vi "Strings to Helium Configuration.vi"(10 "Thresholds":string[][](array[string]), 11 "Timings":string[][](array[string])) -> (2 "Thresholds":T1[](array[typedef]), 3 "Timings":T2[](array[typedef]))   [LabVIEW 2015]
uses:
  Tests/Controls/Test Timing.ctl
  Tests/Controls/Helium Thresholds.ctl
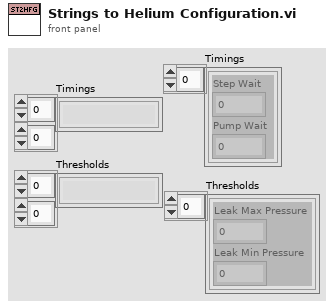
[diagram p1: front panel]
types:
  T1 = typedef "Helium Thresholds.ctl" = cluster{"Leak Max Pressure":dbl, "Leak Min Pressure":dbl}
  T2 = typedef "Test Timing.ctl" = cluster{"Step Wait":dbl, "Pump Wait":dbl}
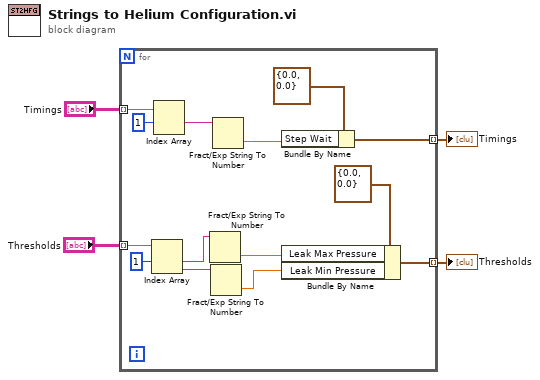
[diagram p0: block diagram]
diagram:
  n1 = for {
    tunnel: "Timings" -> [w18] mode=indexing
    tunnel: "Thresholds" -> [w14] mode=indexing
    tunnel: [w8] -> w2 mode=indexing
    tunnel: [w7] -> w1 mode=indexing
    n2 = Index Array(array=w14, index #1=1 ("index")) -> (element #1=w12:string, element #2=w11:string)  [unwired: 1 in]
    n3 = Index Array(array=w18, index #1=1 ("index")) -> (element #1=w16:string)  [unwired: 1 in, 1 out]
    n4 = Fract/Exp String To Number(string=w12) -> (number=w10:dbl)  [unwired: 3 in, 1 out]
    n5 = Fract/Exp String To Number(string=w11) -> (number=w9:dbl)  [unwired: 3 in, 1 out]
    n6 = Fract/Exp String To Number(string=w16) -> (number=w15:dbl)  [unwired: 3 in, 1 out]
    n7 = Bundle By Name(cluster=T2 {"Step Wait"=0.0, "Pump Wait"=0.0} ("Timing"), "Step Wait"=w15) -> (w8:T2)
    n8 = Bundle By Name(cluster=T1 {"Leak Max Pressure"=0.0, "Leak Min Pressure"=0.0} ("Helium Thresholds"), "Leak Max Pressure"=w10, "Leak Min Pressure"=w9) -> (w7:T1)
  }
  "Timings" <- w2
  "Thresholds" <- w1
